vi "Open UI.vi"(11 "Open UI Msg in":refnum<class "Open UI Msg.lvclass">) -> (0 "error out":errorcluster, 3 "Open UI Msg out":refnum<class "Open UI Msg.lvclass">)   [LabVIEW 2021, in "Open UI.lvlib" / "Open UI Msg.lvclass"]
uses:
  Open UI Msg.lvclass
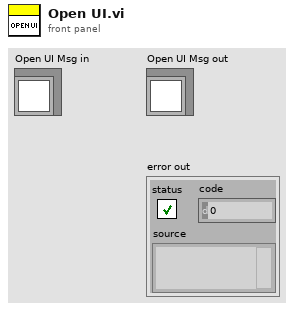
[diagram p1: front panel]
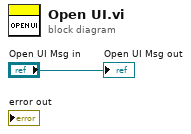
[diagram p0: block diagram]
diagram:
  "Open UI Msg out" <- "Open UI Msg in"
